vi "Build Evaluation String.vi"(6 "VI Path":path, 7 "Assert Scripting Configuration":T1={"Assert Name"="", "Comment"="", "Numeric Operation"="", "Type"=enum."Double Float", "String Operation"="", "DBL Comparison Value 1"=0.0, "DBL Comparison Value 2"=0.0, "I32 Comparison Value 1"=0, "I32 Comparison Value 2"=0, "Creator"="", "Creation Timestamp"=timestamp(0 s since 1904-01-01), "String Comparison Value"="", "Description"="", "Default Failure Action"=enum."None", "Boolean Comparison Value"=FALSE, "I8 Comparison Value 1"=0, "I8 Comparison Value 2"=0, "I16 Comparison Value 1"=0, "I16 Comparison Value 2"=0, "I64 Comparison Value 1"=0, "I64 Comparison Value 2"=0, "U8 Comparison Value 1"=0, "U8 Comparison Value 2"=0, "U16 Comparison Value 1"=0, "U16 Comparison Value 2"=0, "U32 Comparison Value 1"=0, "U32 Comparison Value 2"=0, "U64 Comparison Value 1"=0, "U64 Comparison Value 2"=0, "EXT Comparison Value 1"=0.0, "EXT Comparison Value 2"=0.0, "SGL Comparison Value 1"=0.0, "SGL Comparison Value 2"=0.0}, 8 "error in (no error)":errorcluster) -> (0 "error out":errorcluster, 2 "Evaluation String":string)   [LabVIEW 2016]
doc: "Builds up an evaluation string based on the input parameters specified and applies it to the new assert test vi."
uses:
  Assert Scripting Configuration.ctl
  <vilib>/Utility/Data Type/Type Definitions/Data Type.ctl
  <vilib>/Utility/Data Type/NI_Data Type.lvlib
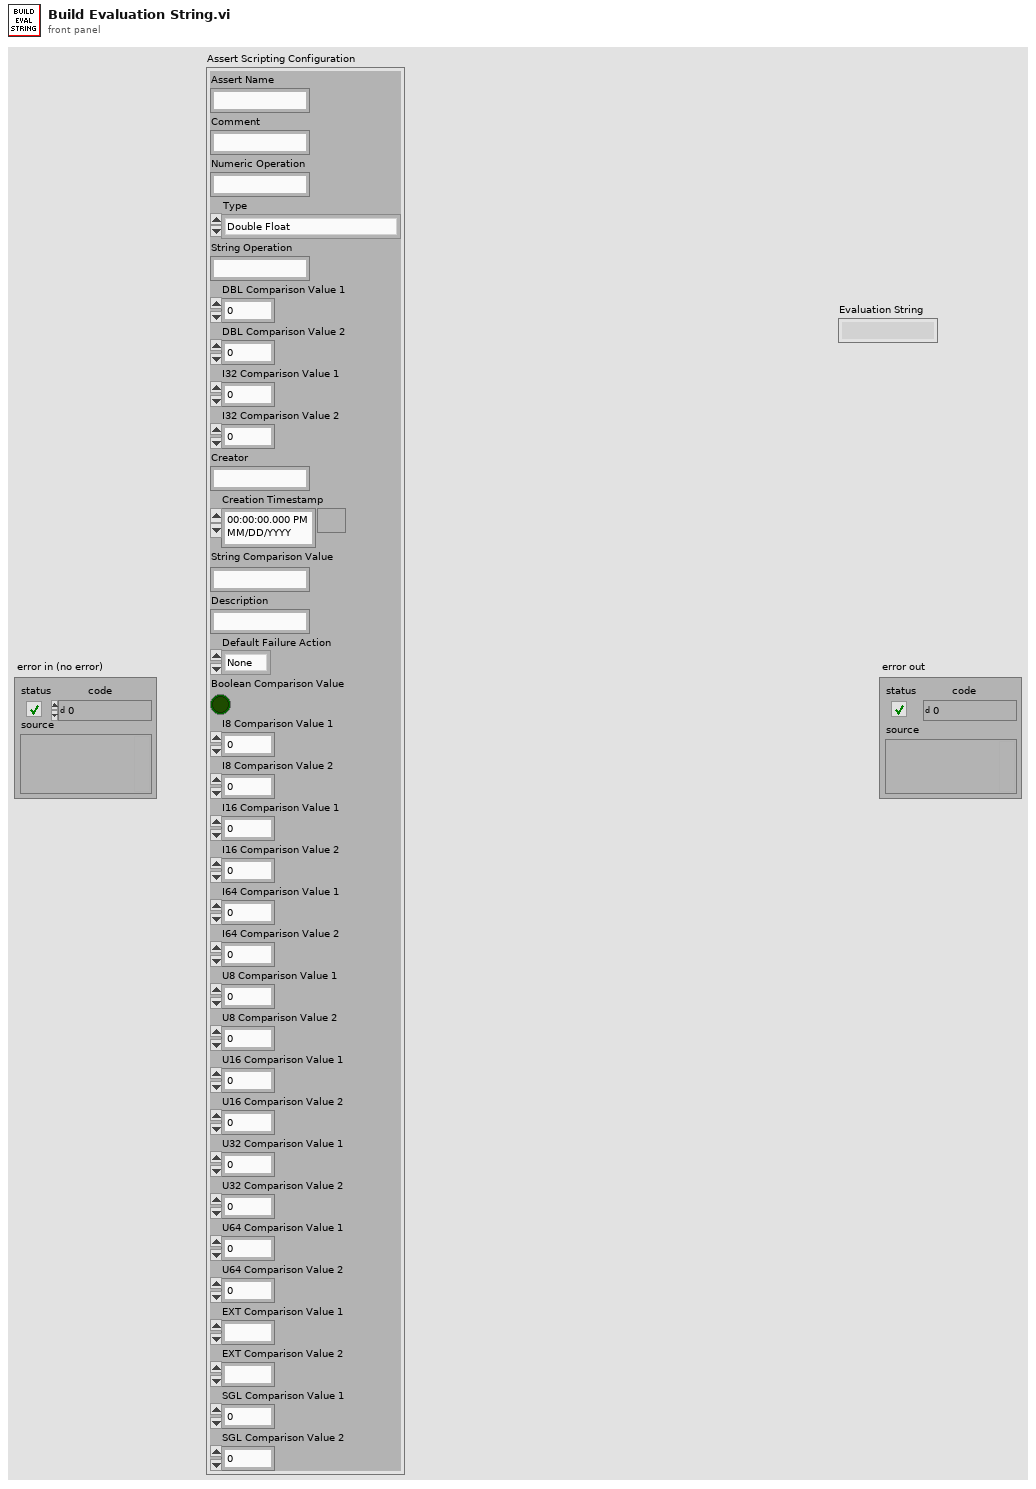
[diagram p1: front panel]
types:
  T1 = typedef "Assert Scripting Configuration.ctl" = cluster{"Assert Name":string, "Comment":string, "Numeric Operation":string, "Type":T2, "String Operation":string, "DBL Comparison Value 1":dbl, "DBL Comparison Value 2":dbl, "I32 Comparison Value 1":i32, "I32 Comparison Value 2":i32, "Creator":string, "Creation Timestamp":timestamp, "String Comparison Value":string, "Description":string, "Default Failure Action":enum16{"None", "Log To File", "Pause Execution", "Abort Execution"}, "Boolean Comparison Value":bool, "I8 Comparison Value 1":i8, "I8 Comparison Value 2":i8, "I16 Comparison Value 1":i16, "I16 Comparison Value 2":i16, "I64 Comparison Value 1":i64, "I64 Comparison Value 2":i64, "U8 Comparison Value 1":u8, "U8 Comparison Value 2":u8, "U16 Comparison Value 1":u16, "U16 Comparison Value 2":u16, "U32 Comparison Value 1":u32, "U32 Comparison Value 2":u32, "U64 Comparison Value 1":u64, "U64 Comparison Value 2":u64, "EXT Comparison Value 1":ext, "EXT Comparison Value 2":ext, "SGL Comparison Value 1":sgl, "SGL Comparison Value 2":sgl}
  T2 = typedef "NI_Data Type.lvlib/Data Type.ctl" = enum8{"Invalid Type", "Void", "I8", "I16", "I32", "I64", "U8", "U16", "U32", "U64", "Single Float", "Double Float", "Extended Float", "Single Complex", "Double Complex", "Extended Complex", "Enum U8", "Enum U16", "Enum U32", "Enum U64", "Single Float With Unit", "Double Float With Unit", "Extended Float With Unit", "Single Complex with Unit", "Double Complex with Unit", "Extended Complex with Unit", "Boolean", "String", "Path", "Picture", "Tag", "Array", "Cluster", "Variant", "LV Variant", "Waveform", "Timestamp", "Digital Waveform", "Digital Data", "ExpressData", "Refnum", "External Data", "VI", "Poly VI", "LabVIEW Class Instance", "Fixed Point"}
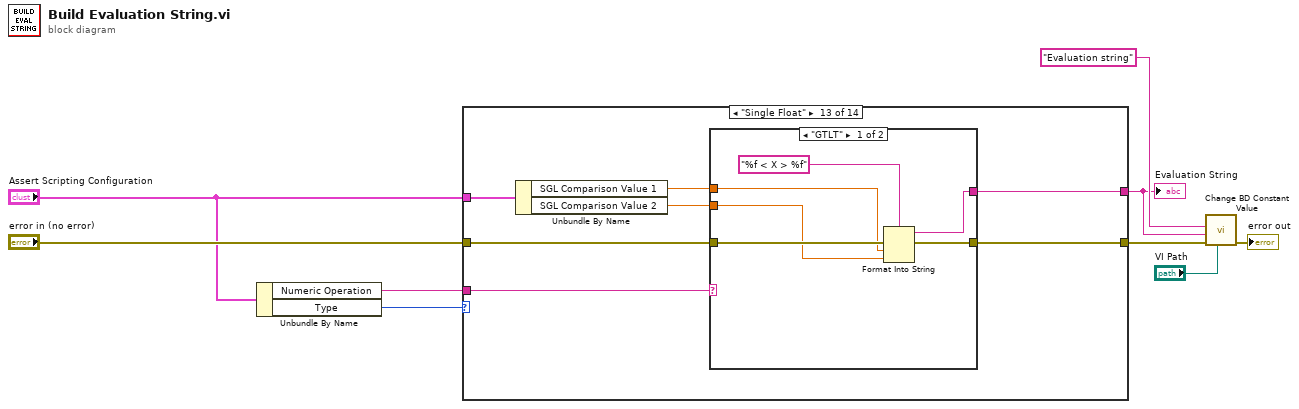
[diagram p0: block diagram]
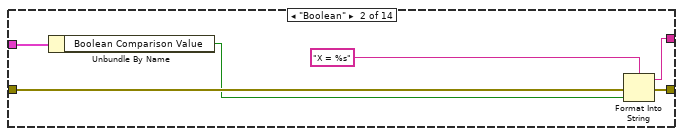
[diagram p3: hidden frame]
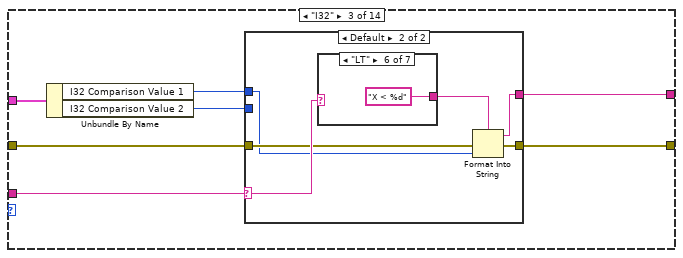
[diagram p4: hidden frame]
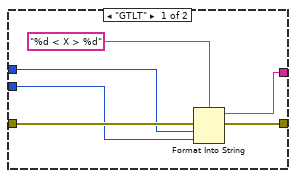
[diagram p5: hidden frame]
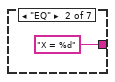
[diagram p7: hidden frame]
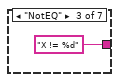
[diagram p8: hidden frame]
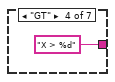
[diagram p9: hidden frame]
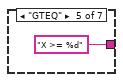
[diagram p10: hidden frame]
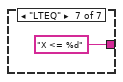
[diagram p11: hidden frame]
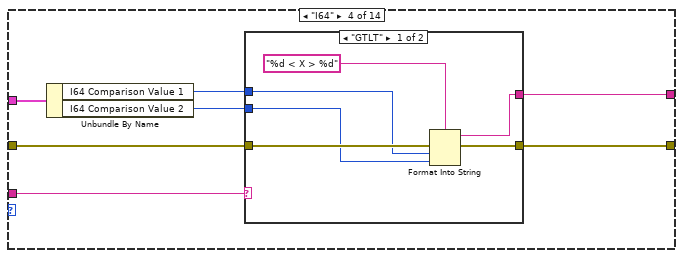
[diagram p12: hidden frame]
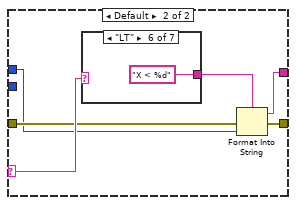
[diagram p13: hidden frame]
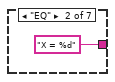
[diagram p15: hidden frame]
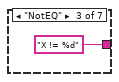
[diagram p16: hidden frame]
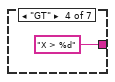
[diagram p17: hidden frame]
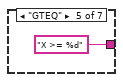
[diagram p18: hidden frame]
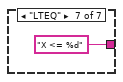
[diagram p19: hidden frame]
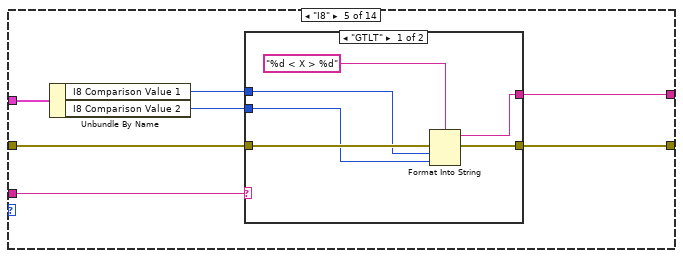
[diagram p20: hidden frame]
diagram:
  n1 = Unbundle By Name("Assert Scripting Configuration") -> ("Numeric Operation"=w7:string, "Type"=w8:T2)
  n2 = case shown="\"Single Float\"" w8 {
    tunnel: w7 -> [_ _ w23 w48 w73 w98 w123 w148 w173 w198 w223 w248 w273 _]
    tunnel: [_ w15 w22 w47 w72 w97 w122 w147 w172 w197 w222 w247 w272 w295] -> w5
    tunnel: "error in (no error)" -> [w10 w14 w21 w46 w71 w96 w121 w146 w171 w196 w221 w246 w271 w298]
    tunnel: [w10 w13 w20 w45 w70 w95 w120 w145 w170 w195 w220 w245 w270 w297] -> w4
    tunnel: "Assert Scripting Configuration" -> [_ w12 w19 w44 w69 w94 w119 w144 w169 w194 w219 w244 w269 w294]
    frame Default {
    }
    frame "Boolean" {
      n3 = Unbundle By Name(w12) -> ("Boolean Comparison Value"=w11:bool)
      n4 = Format Into String(format string="X = %s", error in=w14, w11) -> (resulting string=w15:string, error out=w13:errorcluster)  [unwired: 1 in]
    }
    frame "I32" {
      n5 = Unbundle By Name(w19) -> ("I32 Comparison Value 1"=w18:i32, "I32 Comparison Value 2"=w17:i32)
      n6 = case shown="Default" w23 {
        selector: w23 -> [_ w35]
        tunnel: [w28 w33] -> w22
        tunnel: w21 -> [w27 w32]
        tunnel: [w26 w31] -> w20
        tunnel: w18 -> [w25 w30]
        tunnel: w17 -> [w24 _]
        frame "GTLT" {
          n7 = Format Into String(format string="%d < X > %d", error in=w27, w25, w24) -> (resulting string=w28:string, error out=w26:errorcluster)  [unwired: 1 in]
        }
        frame Default {
          n8 = case shown="\"LT\"" w35 {
            tunnel: [_ "X = %d" "X != %d" "X > %d" "X >= %d" "X < %d" "X <= %d"] -> w34
            frame Default {
            }
            frame "EQ" {
            }
            frame "NotEQ" {
            }
            frame "GT" {
            }
            frame "GTEQ" {
            }
            frame "LT" {
            }
            frame "LTEQ" {
            }
          }
          n9 = Format Into String(format string=w34, error in=w32, w30) -> (resulting string=w33:string, error out=w31:errorcluster)  [unwired: 1 in]
        }
      }
    }
    frame "I64" {
      n10 = Unbundle By Name(w44) -> ("I64 Comparison Value 1"=w43:i64, "I64 Comparison Value 2"=w42:i64)
      n11 = case shown="\"GTLT\"" w48 {
        selector: w48 -> [_ w60]
        tunnel: [w53 w58] -> w47
        tunnel: w46 -> [w52 w57]
        tunnel: [w51 w56] -> w45
        tunnel: w43 -> [w50 w55]
        tunnel: w42 -> [w49 _]
        frame "GTLT" {
          n12 = Format Into String(format string="%d < X > %d", error in=w52, w50, w49) -> (resulting string=w53:string, error out=w51:errorcluster)  [unwired: 1 in]
        }
        frame Default {
          n13 = case shown="\"LT\"" w60 {
            tunnel: [_ "X = %d" "X != %d" "X > %d" "X >= %d" "X < %d" "X <= %d"] -> w59
            frame Default {
            }
            frame "EQ" {
            }
            frame "NotEQ" {
            }
            frame "GT" {
            }
            frame "GTEQ" {
            }
            frame "LT" {
            }
            frame "LTEQ" {
            }
          }
          n14 = Format Into String(format string=w59, error in=w57, w55) -> (resulting string=w58:string, error out=w56:errorcluster)  [unwired: 1 in]
        }
      }
    }
    frame "I8" {
      n15 = Unbundle By Name(w69) -> ("I8 Comparison Value 1"=w68:i8, "I8 Comparison Value 2"=w67:i8)
      n16 = case shown="\"GTLT\"" w73 {
        selector: w73 -> [_ w85]
        tunnel: [w78 w83] -> w72
        tunnel: w71 -> [w77 w82]
        tunnel: [w76 w81] -> w70
        tunnel: w68 -> [w75 w80]
        tunnel: w67 -> [w74 _]
        frame "GTLT" {
          n17 = Format Into String(format string="%d < X > %d", error in=w77, w75, w74) -> (resulting string=w78:string, error out=w76:errorcluster)  [unwired: 1 in]
        }
        frame Default {
          n18 = case shown="\"LT\"" w85 {
            tunnel: [_ "X = %d" "X != %d" "X > %d" "X >= %d" "X < %d" "X <= %d"] -> w84
            frame Default {
            }
            frame "EQ" {
            }
            frame "NotEQ" {
            }
            frame "GT" {
            }
            frame "GTEQ" {
            }
            frame "LT" {
            }
            frame "LTEQ" {
            }
          }
          n19 = Format Into String(format string=w84, error in=w82, w80) -> (resulting string=w83:string, error out=w81:errorcluster)  [unwired: 1 in]
        }
      }
    }
    frame "I16" {
      n20 = Unbundle By Name(w94) -> ("I16 Comparison Value 1"=w93:i16, "I16 Comparison Value 2"=w92:i16)
      n21 = case shown="\"GTLT\"" w98 {
        selector: w98 -> [_ w110]
        tunnel: [w103 w108] -> w97
        tunnel: w96 -> [w102 w107]
        tunnel: [w101 w106] -> w95
        tunnel: w93 -> [w100 w105]
        tunnel: w92 -> [w99 _]
        frame "GTLT" {
          n22 = Format Into String(format string="%d < X > %d", error in=w102, w100, w99) -> (resulting string=w103:string, error out=w101:errorcluster)  [unwired: 1 in]
        }
        frame Default {
          n23 = case shown="\"LT\"" w110 {
            tunnel: [_ "X = %d" "X != %d" "X > %d" "X >= %d" "X < %d" "X <= %d"] -> w109
            frame Default {
            }
            frame "EQ" {
            }
            frame "NotEQ" {
            }
            frame "GT" {
            }
            frame "GTEQ" {
            }
            frame "LT" {
            }
            frame "LTEQ" {
            }
          }
          n24 = Format Into String(format string=w109, error in=w107, w105) -> (resulting string=w108:string, error out=w106:errorcluster)  [unwired: 1 in]
        }
      }
    }
    frame "U8" {
      n25 = Unbundle By Name(w119) -> ("U8 Comparison Value 1"=w118:u8, "U8 Comparison Value 2"=w117:u8)
      n26 = case shown="\"GTLT\"" w123 {
        selector: w123 -> [_ w135]
        tunnel: [w128 w133] -> w122
        tunnel: w121 -> [w127 w132]
        tunnel: [w126 w131] -> w120
        tunnel: w118 -> [w125 w130]
        tunnel: w117 -> [w124 _]
        frame "GTLT" {
          n27 = Format Into String(format string="%d < X > %d", error in=w127, w125, w124) -> (resulting string=w128:string, error out=w126:errorcluster)  [unwired: 1 in]
        }
        frame Default {
          n28 = case shown="\"LT\"" w135 {
            tunnel: [_ "X = %d" "X != %d" "X > %d" "X >= %d" "X < %d" "X <= %d"] -> w134
            frame Default {
            }
            frame "EQ" {
            }
            frame "NotEQ" {
            }
            frame "GT" {
            }
            frame "GTEQ" {
            }
            frame "LT" {
            }
            frame "LTEQ" {
            }
          }
          n29 = Format Into String(format string=w134, error in=w132, w130) -> (resulting string=w133:string, error out=w131:errorcluster)  [unwired: 1 in]
        }
      }
    }
    frame "U16" {
      n30 = Unbundle By Name(w144) -> ("U16 Comparison Value 1"=w143:u16, "U16 Comparison Value 2"=w142:u16)
      n31 = case shown="\"GTLT\"" w148 {
        selector: w148 -> [_ w160]
        tunnel: [w153 w158] -> w147
        tunnel: w146 -> [w152 w157]
        tunnel: [w151 w156] -> w145
        tunnel: w143 -> [w150 w155]
        tunnel: w142 -> [w149 _]
        frame "GTLT" {
          n32 = Format Into String(format string="%d < X > %d", error in=w152, w150, w149) -> (resulting string=w153:string, error out=w151:errorcluster)  [unwired: 1 in]
        }
        frame Default {
          n33 = case shown="\"LT\"" w160 {
            tunnel: [_ "X = %d" "X != %d" "X > %d" "X >= %d" "X < %d" "X <= %d"] -> w159
            frame Default {
            }
            frame "EQ" {
            }
            frame "NotEQ" {
            }
            frame "GT" {
            }
            frame "GTEQ" {
            }
            frame "LT" {
            }
            frame "LTEQ" {
            }
          }
          n34 = Format Into String(format string=w159, error in=w157, w155) -> (resulting string=w158:string, error out=w156:errorcluster)  [unwired: 1 in]
        }
      }
    }
    frame "U32" {
      n35 = Unbundle By Name(w169) -> ("U32 Comparison Value 1"=w168:u32, "U32 Comparison Value 2"=w167:u32)
      n36 = case shown="\"GTLT\"" w173 {
        selector: w173 -> [_ w185]
        tunnel: [w178 w183] -> w172
        tunnel: w171 -> [w177 w182]
        tunnel: [w176 w181] -> w170
        tunnel: w168 -> [w175 w180]
        tunnel: w167 -> [w174 _]
        frame "GTLT" {
          n37 = Format Into String(format string="%d < X > %d", error in=w177, w175, w174) -> (resulting string=w178:string, error out=w176:errorcluster)  [unwired: 1 in]
        }
        frame Default {
          n38 = case shown="\"LT\"" w185 {
            tunnel: [_ "X = %d" "X != %d" "X > %d" "X >= %d" "X < %d" "X <= %d"] -> w184
            frame Default {
            }
            frame "EQ" {
            }
            frame "NotEQ" {
            }
            frame "GT" {
            }
            frame "GTEQ" {
            }
            frame "LT" {
            }
            frame "LTEQ" {
            }
          }
          n39 = Format Into String(format string=w184, error in=w182, w180) -> (resulting string=w183:string, error out=w181:errorcluster)  [unwired: 1 in]
        }
      }
    }
    frame "U64" {
      n40 = Unbundle By Name(w194) -> ("U64 Comparison Value 1"=w193:u64, "U64 Comparison Value 2"=w192:u64)
      n41 = case shown="\"GTLT\"" w198 {
        selector: w198 -> [_ w210]
        tunnel: [w203 w208] -> w197
        tunnel: w196 -> [w202 w207]
        tunnel: [w201 w206] -> w195
        tunnel: w193 -> [w200 w205]
        tunnel: w192 -> [w199 _]
        frame "GTLT" {
          n42 = Format Into String(format string="%d < X > %d", error in=w202, w200, w199) -> (resulting string=w203:string, error out=w201:errorcluster)  [unwired: 1 in]
        }
        frame Default {
          n43 = case shown="\"LT\"" w210 {
            tunnel: [_ "X = %d" "X != %d" "X > %d" "X >= %d" "X < %d" "X <= %d"] -> w209
            frame Default {
            }
            frame "EQ" {
            }
            frame "NotEQ" {
            }
            frame "GT" {
            }
            frame "GTEQ" {
            }
            frame "LT" {
            }
            frame "LTEQ" {
            }
          }
          n44 = Format Into String(format string=w209, error in=w207, w205) -> (resulting string=w208:string, error out=w206:errorcluster)  [unwired: 1 in]
        }
      }
    }
    frame "Double Float" {
      n45 = Unbundle By Name(w219) -> ("DBL Comparison Value 1"=w218:dbl, "DBL Comparison Value 2"=w217:dbl)
      n46 = case shown="Default" w223 {
        selector: w223 -> [_ w235]
        tunnel: [w228 w233] -> w222
        tunnel: w221 -> [w227 w232]
        tunnel: [w226 w231] -> w220
        tunnel: w218 -> [w225 w230]
        tunnel: w217 -> [w224 _]
        frame "GTLT" {
          n47 = Format Into String(format string="%f < X > %f", error in=w227, w225, w224) -> (resulting string=w228:string, error out=w226:errorcluster)  [unwired: 1 in]
        }
        frame Default {
          n48 = case shown="\"EQ\"" w235 {
            tunnel: [_ "X = %f" "X != %f" "X > %f" "X >= %f" "X < %f" "X <= %f"] -> w234
            frame Default {
            }
            frame "EQ" {
            }
            frame "NotEQ" {
            }
            frame "GT" {
            }
            frame "GTEQ" {
            }
            frame "LT" {
            }
            frame "LTEQ" {
            }
          }
          n49 = Format Into String(format string=w234, error in=w232, w230) -> (resulting string=w233:string, error out=w231:errorcluster)  [unwired: 1 in]
        }
      }
    }
    frame "Extended Float" {
      n50 = Unbundle By Name(w244) -> ("EXT Comparison Value 1"=w243:ext, "EXT Comparison Value 2"=w242:ext)
      n51 = case shown="Default" w248 {
        selector: w248 -> [_ w260]
        tunnel: [w253 w258] -> w247
        tunnel: w246 -> [w252 w257]
        tunnel: [w251 w256] -> w245
        tunnel: w243 -> [w250 w255]
        tunnel: w242 -> [w249 _]
        frame "GTLT" {
          n52 = Format Into String(format string="%f < X > %f", error in=w252, w250, w249) -> (resulting string=w253:string, error out=w251:errorcluster)  [unwired: 1 in]
        }
        frame Default {
          n53 = case shown="\"EQ\"" w260 {
            tunnel: [_ "X = %f" "X != %f" "X > %f" "X >= %f" "X < %f" "X <= %f"] -> w259
            frame Default {
            }
            frame "EQ" {
            }
            frame "NotEQ" {
            }
            frame "GT" {
            }
            frame "GTEQ" {
            }
            frame "LT" {
            }
            frame "LTEQ" {
            }
          }
          n54 = Format Into String(format string=w259, error in=w257, w255) -> (resulting string=w258:string, error out=w256:errorcluster)  [unwired: 1 in]
        }
      }
    }
    frame "Single Float" {
      n55 = Unbundle By Name(w269) -> ("SGL Comparison Value 1"=w268:sgl, "SGL Comparison Value 2"=w267:sgl)
      n56 = case shown="\"GTLT\"" w273 {
        selector: w273 -> [_ w285]
        tunnel: [w278 w283] -> w272
        tunnel: w271 -> [w277 w282]
        tunnel: [w276 w281] -> w270
        tunnel: w268 -> [w275 w280]
        tunnel: w267 -> [w274 _]
        frame "GTLT" {
          n57 = Format Into String(format string="%f < X > %f", error in=w277, w275, w274) -> (resulting string=w278:string, error out=w276:errorcluster)  [unwired: 1 in]
        }
        frame Default {
          n58 = case shown="\"GT\"" w285 {
            tunnel: [_ "X = %f" "X != %f" "X > %f" "X >= %f" "X < %f" "X <= %f"] -> w284
            frame Default {
            }
            frame "EQ" {
            }
            frame "NotEQ" {
            }
            frame "GT" {
            }
            frame "GTEQ" {
            }
            frame "LT" {
            }
            frame "LTEQ" {
            }
          }
          n59 = Format Into String(format string=w284, error in=w282, w280) -> (resulting string=w283:string, error out=w281:errorcluster)  [unwired: 1 in]
        }
      }
    }
    frame "String" {
      n60 = Unbundle By Name(w294) -> ("String Operation"=w293:string, "String Comparison Value"=w292:string)
      n61 = case shown="\"EW\"" w293 {
        tunnel: [_ "String = \"%s\"" "String != \"%s\"" "String should contain \"%s\"" "String should not contain \"%s\"" "String start with \"%s\"" "String end with \"%s\""] -> w296
        frame Default {
        }
        frame "EQ" {
        }
        frame "NotEQ" {
        }
        frame "Contains" {
        }
        frame "NotContain" {
        }
        frame "SW" {
        }
        frame "EW" {
        }
      }
      n62 = Format Into String(format string=w296, error in=w298, w292) -> (resulting string=w295:string, error out=w297:errorcluster)  [unwired: 1 in]
    }
  }
  "Evaluation String" <- w5
  n63 = call "Change BD Constant Value.vi"("Assert VI Path"="VI Path", "error in (no error)"=w4, "Data Value"=w5, "Constant Name"="Evaluation string") -> ("error out"=→"error out":errorcluster)  [unwired: 7 in]
